vi "RaiseAfterDriveAtDistance-C.vi"(11 "Params":string[][](array[string])) -> ()   [LabVIEW 2018]
uses:
  Framework/Robot Global Data.vi
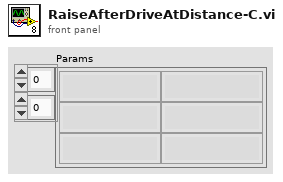
[diagram p1: front panel]
types:
  T1 = typedef "Command Status Info.ctl" = cluster{"Name":string, "Status":T2, "notifier out":T3}
  T2 = typedef "Completion Status.ctl" = enum16{"Successful", "Aborted", "Incomplete"}
  T3 = typedef "Completion Notifier.ctl" = refnum<notifier>
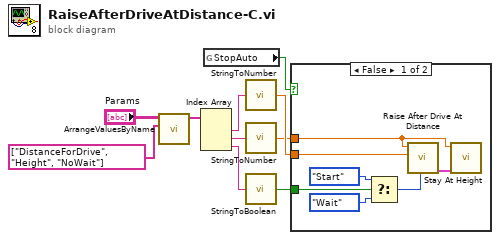
[diagram p0: block diagram]
diagram:
  n1 = call "ArrangeValuesByName.vi"("Names"=string[] ["DistanceForDrive", "Height", "NoWait"], "Names/Values in"="Params") -> ("Values Out"=w4:string[])  [unwired: 9 in]
  n2 = Index Array(array=w4) -> (element #1=w3:string, element #2=w2:string, element #3=w1:string)  [unwired: 3 in]
  n3 = global read "Robot Global Data.vi" "StopAuto"() -> (w10:bool)
  n4 = call "StringToNumber.vi"("String"=w3) -> ("Output"=w9:dbl)
  n5 = call "StringToNumber.vi"("String"=w2) -> ("Output"=w8:dbl)
  n6 = call "StringToBoolean.vi"("String"=w1) -> ("Output"=w7:bool)
  n7 = case shown="False" w10 {
    tunnel: w9 -> [w13 _]
    tunnel: w8 -> [w11 _]
    tunnel: w7 -> [w15 _]
    frame False {
      n8 = Select(t=enum16{"Start", "Wait"}."Start" ("Synchronization"), s=w15, f=enum16{"Start", "Wait"}."Wait" ("Synchronization")) -> (s? t:f=w14:enum16{"Start", "Wait"})
      n9 = call "Raise After Drive At Distance.vi"("Synchronization"=w14, "DistanceForDrive"=w13, "Height"=w11) -> ("Command Info Out"=w12:T1)  [unwired: 8 in]
      n10 = call "Stay At Height.vi"("Command Info In"=w12, "Height"=w11) -> ()  [unwired: 9 in, 1 out]
    }
    frame True {
    }
  }
